vi "OBD_speed.vi"(8 "error in":errorcluster, 11 "Cluster input":T1) -> (0 "error out":errorcluster, 3 "Output cluster":T1)   [LabVIEW 2020]
doc: "The Advanced Serial Read and Write example performs a Serial Port Read, a Serial Port Write, or a combination of these actions while setting some advanced serial features like buffer size, termination characters, and XON/XOFF flow control. The user selects the actions (read or write) on the front panel. If both are selected, the VI will write the data first, read the data and then close the VISA session that is opened to the port. \n\nThe parameters set for the serial port must match the parameters of the connected instrument or device. In this example, the bytes to read parameter specifies the number of bytes that the serial port reads. If there were more bytes at the port than the number specified in bytes to read, those bytes would not be read. Also, if you specify to read more bytes than the number of bytes actually read, you might receive a timeout error message.\n\nINSTRUCTIONS:\n1) Select the serial resource and configuration parameters (baud rate, data bits, parity, stop bits, flow control).\n2) Termination character can be enabled and set. Also, set the required input buffer size prior to running the example.\n3) Select the operations to be performed. \n4) Connect the serial port to your device. If no device is available, perform a loopback test by doing one of the following. Short pins 2 and 3 on a RS-232 cable or short pin 4 to pin 8 and pin 5 to pin 9 on a RS-485/422 cable. \n5) Run the VI to see the data read. (The \"read string\" will match the \"string to write\" if a loopback test was performed.)\n\nThis example exposes several advanced features that you may need for your application. Not all applications need all the features shown in this example. The input buffer size is likely an important setting that you want to control in your application. This example expands upon the flow control option for XON and XOFF, allowing the user to choose those control characters. The timeout parameter has been brought to the front panel so a user can specify the time period the VISA Read will wait for the number of bytes to read before timing out. Also, the user has several controls for the termination character, which is discussed later.\n\nNote that you can press the write and read buttons and change the bytes to read parameters on the fly, while the example is running. However, you must stop the example to change the other configuration parameters after the example has started running, and then run again.\n\nSet the I/O buffer size slightly higher the amount of data you expect to receive. This is very important for applications that don't use flow control, as you may lose characters if the receive buffer overflows.\n\nSetting the timeout period ensures that the operation returns with a timeout error if the operation cannot be performed in the specified time period. \n\nSome devices require a termination character in order to identify the end of command strings. Some devices send a termination character to signify the end of data to be read. \n\nThis example shows how you can end the Read operation once a termination character is detected in the buffer and/or append a termination character at the end of the Write data. To enable the Read to end on a termination character, use the VISA Configure Serial Port or use the VISA Properties Serial End Mode for Reads, Termination Character Enable, and Termination Character. To end the Write with a termination character, use the VISA Properties Serial End Mode for Writes, the Send End Enable, and Termination Character. In this example, the same termination character is used for both the Read and the Write. You can specify two different characters for your application, if desired.\n\nYour application may require specific characters for the XON/XOFF Flow Control. You can specify these characters with the VISA Properties Flow Control XOFF Character and Flow Control XON Character. Note that if the standard XON and XOFF characters are used, then decimal 17 and 19 are unavailable for data values. Remember that using flow control and setting an adequate buffer size allow you to prevent buffer overflows."
uses:
  controls/StateMachineVariables.ctl
  <vilib>/vision/Avi.llb/IMAQ AVI2 Refnum.ctl
  <vilib>/userDefined/High Color/IMAQdx.ctl
  <vilib>/vision/Deep Learning.llb/IMAQ DL Model Refnum.ctl
  <vilib>/vision/Image Controls.llb/IMAQ Image.ctl
  terminal_test.vi
panel:
  out "Messages":string
  out "Speed (km/h)":u32(graph)
  out "Speed (km/h)":u32
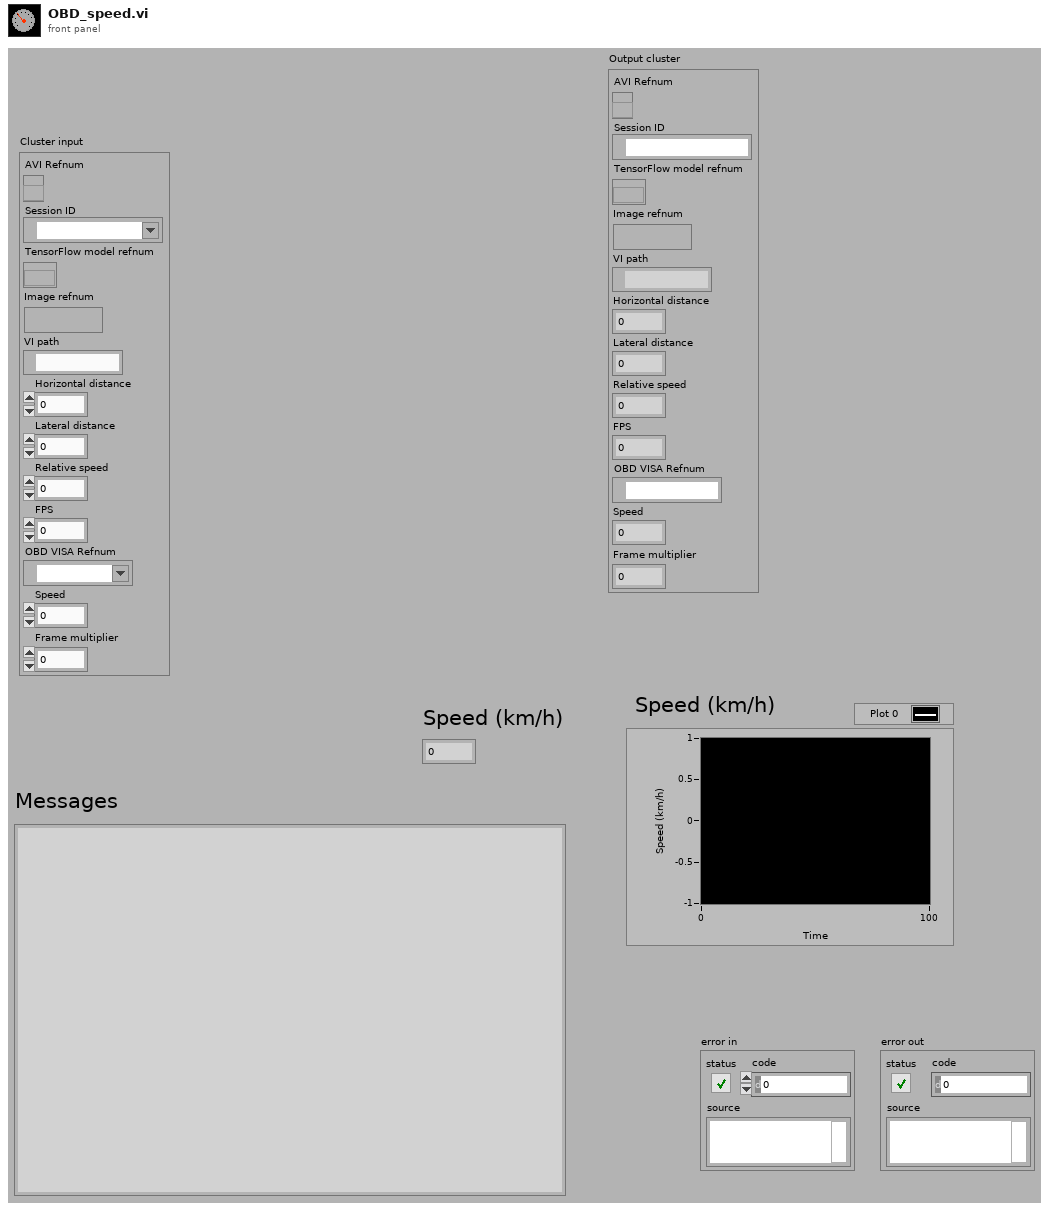
[diagram p1: front panel]
types:
  T1 = typedef "StateMachineVariables.ctl" = cluster{"AVI Refnum":T2, "Session ID":T3, "TensorFlow model refnum":T4, "Image refnum":T5, "VI path":path, "Horizontal distance":dbl, "Lateral distance":dbl, "Relative speed":dbl, "FPS":dbl, "OBD VISA Refnum":refnum<visa-resource-name>, "Speed":dbl, "Frame multiplier":u32}
  T2 = typedef "IMAQ AVI2 Refnum.ctl" = refnum<k20>
  T3 = typedef "IMAQdx.ctl" = refnum<k21>
  T4 = typedef "IMAQ DL Model Refnum.ctl" = refnum<k20>
  T5 = typedef "IMAQ Image.ctl" = refnum<image>
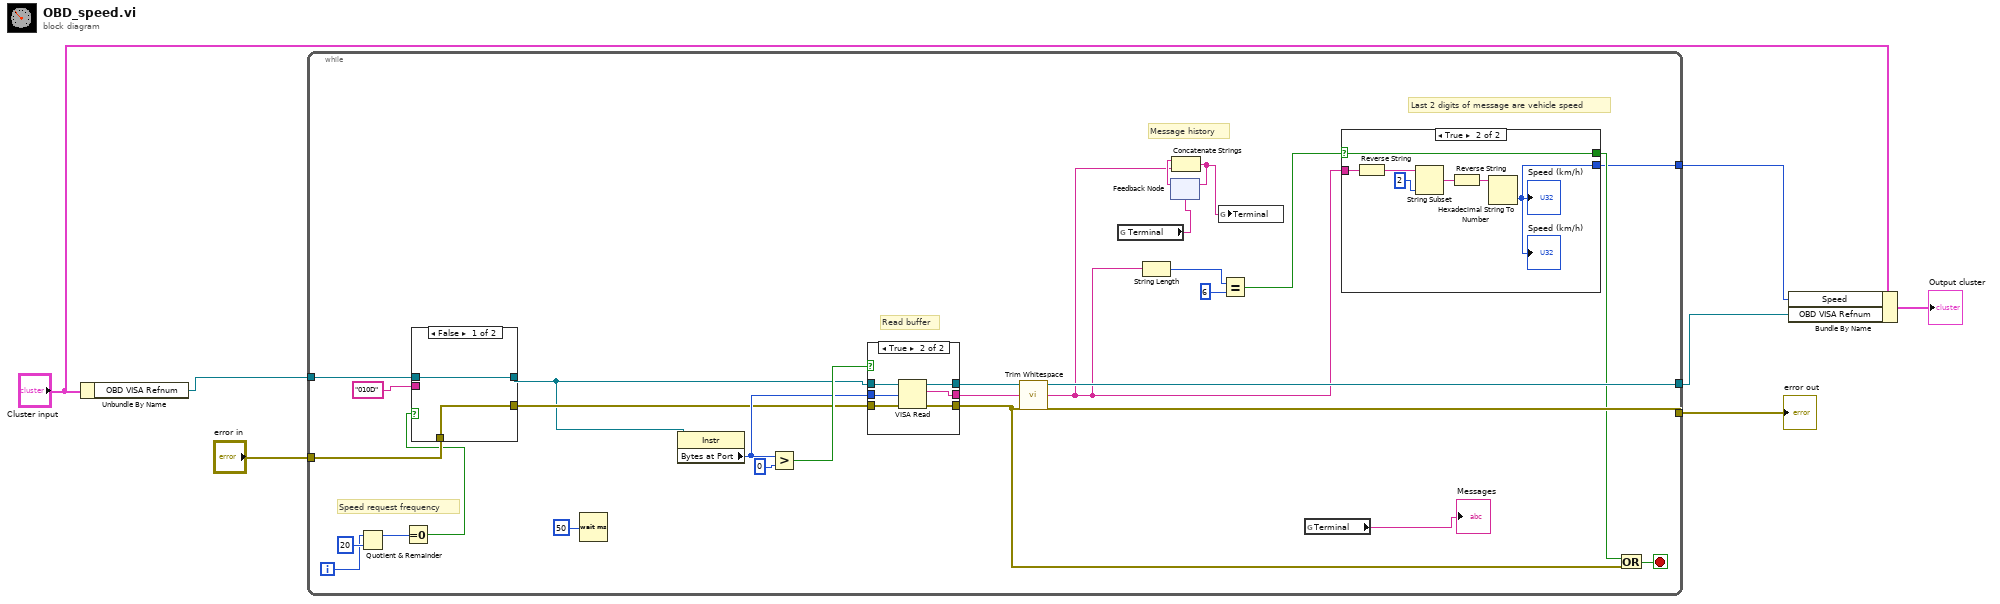
[diagram p0: block diagram]
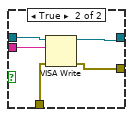
[diagram p2: hidden frame]
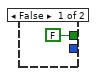
[diagram p3: hidden frame]
diagram:
  n1 = Unbundle By Name("Cluster input") -> ("OBD VISA Refnum"=w1:refnum<visa-resource-name>)
  n2 = while {
    tunnel: [w32] -> w5
    tunnel: [w21] -> w7
    tunnel: [w18] -> w3
    tunnel: "error in" -> [w16]
    tunnel: w1 -> [w15]
    i -> [w9]
    stop <- w26 stop-if-true
    # "Speed request frequency"
    # "Read buffer"
    # "Last 2 digits of message are vehicle speed"
    # "Message history"
    n3 = Quotient & Remainder(x=w9, y=20) -> (x-y*floor(x/y)=w10:i32)  [unwired: 1 out]
    n4 = Equal To 0?(x=w10) -> (x = 0?=w8:bool)
    n5 = case shown="False" w8 {
      tunnel: w16 -> [w35 w41]
      tunnel: w15 -> [w36 w40]
      tunnel: [w35 w39] -> w14
      tunnel: "010D" ("String") -> [_ w38]
      tunnel: [w36 w37] -> w12
      frame False {
      }
      frame True {
        n6 = VISA Write(VISA resource name=w40, write buffer=w38, error in (no error)=w41) -> (VISA resource name out=w37:refnum<visa-resource-name>, error out=w39:errorcluster)  [unwired: 1 out]
      }
    }
    n7 = Wait (ms)(milliseconds to wait=u32 50) -> ()  [unwired: 1 out]
    n8 = property class="Instr"(reference=w12) -> ("Bytes at Port"=w31:u32)  [unwired: 1 in, 2 out]
    n9 = Greater?(x=w31, y=u32 0) -> (0:w33:bool)
    n10 = case shown="True" w33 {
      tunnel: [w50 w57] -> w21
      tunnel: [w51 w56] -> w32
      tunnel: w14 -> [w50 w55]
      tunnel: w12 -> [w51 w54]
      tunnel: [_ w53] -> w29
      tunnel: w31 -> [_ w52]
      frame False {
      }
      frame True {
        n11 = VISA Read(VISA resource name=w54, byte count=w52, error in (no error)=w55) -> (VISA resource name out=w56:refnum<visa-resource-name>, read buffer=w53:string, error out=w57:errorcluster)  [unwired: 1 out]
      }
    }
    n12 = call <vilib>:"Trim Whitespace.vi"("string"=w29) -> ("trimmed string"=w23:string)  [unwired: 1 in]
    n13 = global read "terminal_test.vi" "Terminal"() -> (w28:string)
    n14 = String Length(string=w23) -> (length=w25:i32)
    n15 = feedback #1(w28) -> (w30:string)
    n16 = Concatenate Strings(w30, w23) -> (w27:string)
    n17 = feedback-in #1(w27) -> ()
    n18 = global write "terminal_test.vi" "Terminal"(w27) -> ()
    n19 = Equal?(x=w25, y=6) -> (x = y?=w22:bool)
    n20 = global read "terminal_test.vi" "Terminal"() -> (→"Messages":string)
    n21 = case shown="True" w22 {
      selector: w22 -> [_ w44]
      tunnel: w23 -> [_ w47]
      tunnel: [FALSE w44] -> w20
      tunnel: [_ w43] -> w18
      frame False {
      }
      frame True {
        n22 = Reverse String(1:w47) -> (0:w49:string)
        n23 = String Subset(string=w49, length (rest)=2 ("length (rest)")) -> (substring=w46:string)  [unwired: 1 in]
        n24 = Reverse String(1:w46) -> (0:w45:string)
        n25 = Hexadecimal String To Number(string=w45) -> (number=w43:u32)  [unwired: 2 in, 1 out]
        "Speed (km/h)" <- w43
        "Speed (km/h)" <- w43
      }
    }
    n26 = Or(x=w20, y=w21) -> (x .or. y?=w26:bool)
  }
  "error out" <- w7
  n27 = Bundle By Name(cluster="Cluster input", "Speed"=w3, "OBD VISA Refnum"=w5) -> (→"Output cluster":T1)
